vi "LED and Push Button.vi"() -> ()   [LabVIEW 2016]
uses:
  <vilib>/rvi/Emulation/niFpgaGetClockAttributes.vi
  <vilib>/rvi/Emulation/niFpgaSctlEmulationGetInTimedLoop.vi
  <vilib>/rvi/Emulation/niFpgaEmulationReportErrorSimple.vi
  <vilib>/rvi/eio/common/nirviEmuTemplateMethod_errors.vi
  <vilib>/rvi/Emulation/niFpgaCriticalErrorInLSC.vi
  <vilib>/eio/EIONode/EIONode.xnode
panel:
  out "LED Set 2":bool
  out "LED Set1":bool
  in  "stop":bool
  out "Switch":bool
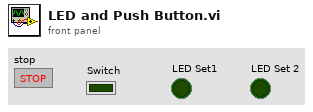
[diagram p1: front panel]
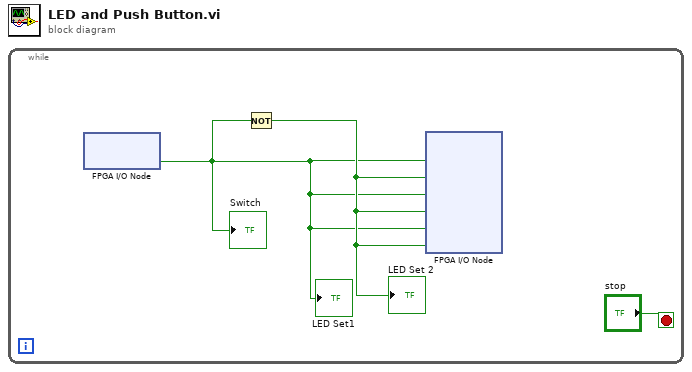
[diagram p0: block diagram]
diagram:
  n1 = while {
    stop <- "stop" stop-if-true
    n2 = xnode "FPGA I/O Node"() -> ("DIO13"=w1:bool)  [unwired: 1 in, 1 out]
    "Switch" <- w1
    "LED Set1" <- w1
    n3 = Not(x=w1) -> (.not. x?=w2:bool)
    "LED Set 2" <- w2
    n4 = xnode "FPGA I/O Node"("DIO4"=w1, "DIO5"=w2, "DIO6"=w1, "DIO7"=w2, "DIO8"=w1, "DIO9"=w2) -> ()  [unwired: 6 in, 6 out]
  }
